vi "Runner_Enter.vi"(8 "error in":errorcluster) -> (0 "error out":errorcluster, 3 "Runner's Data OUT":T1)   [LabVIEW 2025]
uses:
  Controls/Runner_Data_Structure.ctl
panel:
  in  "Button":bool
  in  "Runner's Data IN":T1
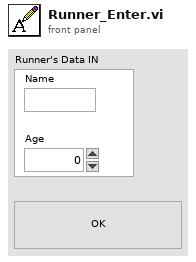
[diagram p1: front panel]
types:
  T1 = typedef "Runner_Data_Structure.ctl" = cluster{"Name":string, "Age":i32}
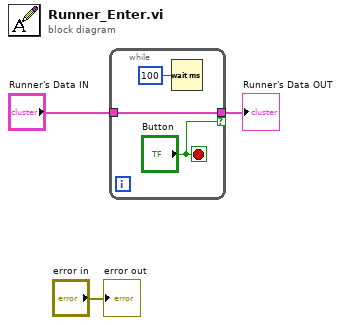
[diagram p0: block diagram]
diagram:
  n1 = while {
    tunnel: "Runner's Data IN" -> [w6]
    tunnel: [w6] -> w2 if="Button"
    stop <- "Button" stop-if-true
    n2 = Wait (ms)(milliseconds to wait=u32 100) -> ()  [unwired: 1 out]
  }
  "Runner's Data OUT" <- w2
  "error out" <- "error in"
